vi "Expand Digital Pattern.vi"(5 "Zoom":refnum<vi>, 7 "Pattern Plot":refnum<vi>, 8 "error in (no error)":errorcluster, 9 "Select Patterns":i32[](array[numeric]), 10 "Rotations":u16, 11 "Patterns":T1[](array[typedef])) -> (0 "error out":errorcluster)   [LabVIEW 2017, in "Engine Simulation Toolkit System Explorer.lvlib"]
uses:
  Engine Simulation Toolkit System Explorer.lvlib
  Digital Pattern.ctl
  Digital Pattern Base.ctl
  Digital Pattern Remove Edge.ctl
  Digital Pattern Add Pulse.ctl
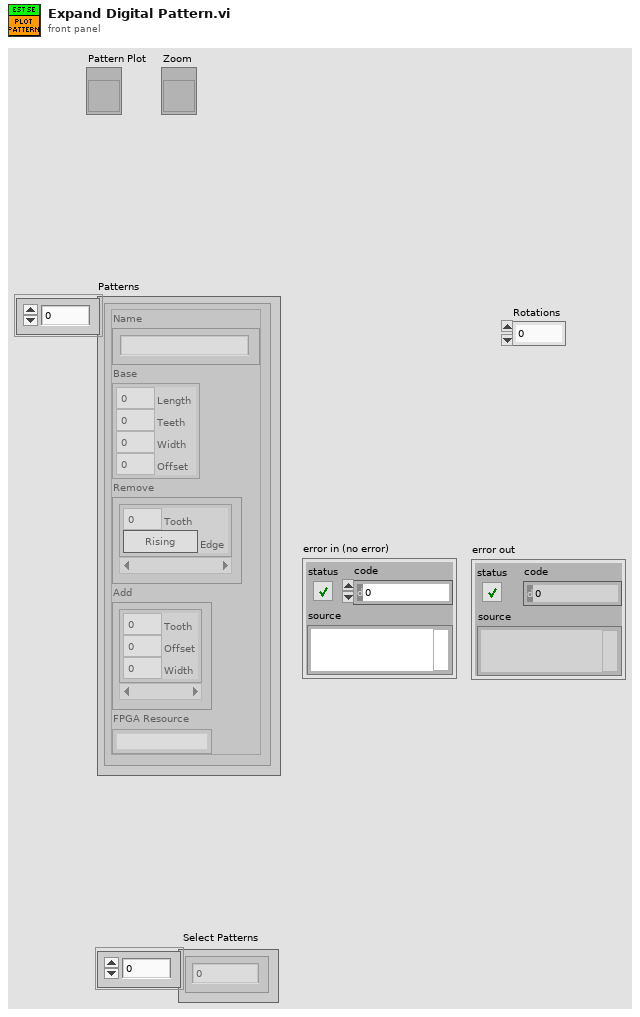
[diagram p1: front panel]
types:
  T1 = typedef "Engine Simulation Toolkit System Explorer.lvlib/Digital Pattern.ctl" = cluster{"Name":string, "Base":T2, "Remove":T3[], "Add":T4[], "FPGA Resource":string}
  T2 = typedef "Engine Simulation Toolkit System Explorer.lvlib/Digital Pattern Base.ctl" = cluster{"Length":dbl, "Teeth":u16, "Width":dbl, "Offset":dbl}
  T3 = typedef "Engine Simulation Toolkit System Explorer.lvlib/Digital Pattern Remove Edge.ctl" = cluster{"Tooth":u16, "Edge":bool}
  T4 = typedef "Engine Simulation Toolkit System Explorer.lvlib/Digital Pattern Add Pulse.ctl" = cluster{"Tooth":u16, "Offset":dbl, "Width":dbl}
  T5 = cluster{"Name":string, "Color":u32, "Style":u8, "Point Style":u8, "Name Visible":bool, "Allow Drag":bool, "Cursor Mode":u32, "Plot":i32, "Index":i32, "Position":cluster{"X":dbl, "Y":dbl}, "X Scale":u32, "Y Scale":u32, "Watch Plots":i32[], "Watch All Plots":bool, "Plot Area":i32, "Label Offset":cluster{"X":dbl, "Y":dbl}}
  T6 = cluster{"Name":string, "Color":u32, "Style":u8, "Point Style":u8, "Name Visible":bool, "Allow Drag":bool, "Cursor Mode":u32, "Plot":i32, "Index":i32, "Position":cluster{"X":dbl, "Y":dbl}, "X Scale":u32, "Y Scale":u32, "Watch Plots":i32[], "Watch All Plots":bool, "Plot Area":i32, "Label Offset":cluster{"X":dbl, "Y":dbl}}[]
  T7 = typedef "LVCursorListTypeDef.ctl" = cluster{"Name":string, "Color":u32, "Style":u8, "Point Style":u8, "Name Visible":bool, "Allow Drag":bool, "Cursor Mode":u32, "Plot":i32, "Index":i32, "Position":cluster{"X":dbl, "Y":dbl}, "X Scale":u32, "Y Scale":u32, "Watch Plots":i32[], "Watch All Plots":bool, "Plot Area":i32, "Label Offset":cluster{"X":dbl, "Y":dbl}}[]
  T8 = typedef "Engine Simulation Toolkit System Explorer.lvlib/Digital Pattern Expanded.ctl" = cluster{"X":dbl[], "Y":dbl[]}
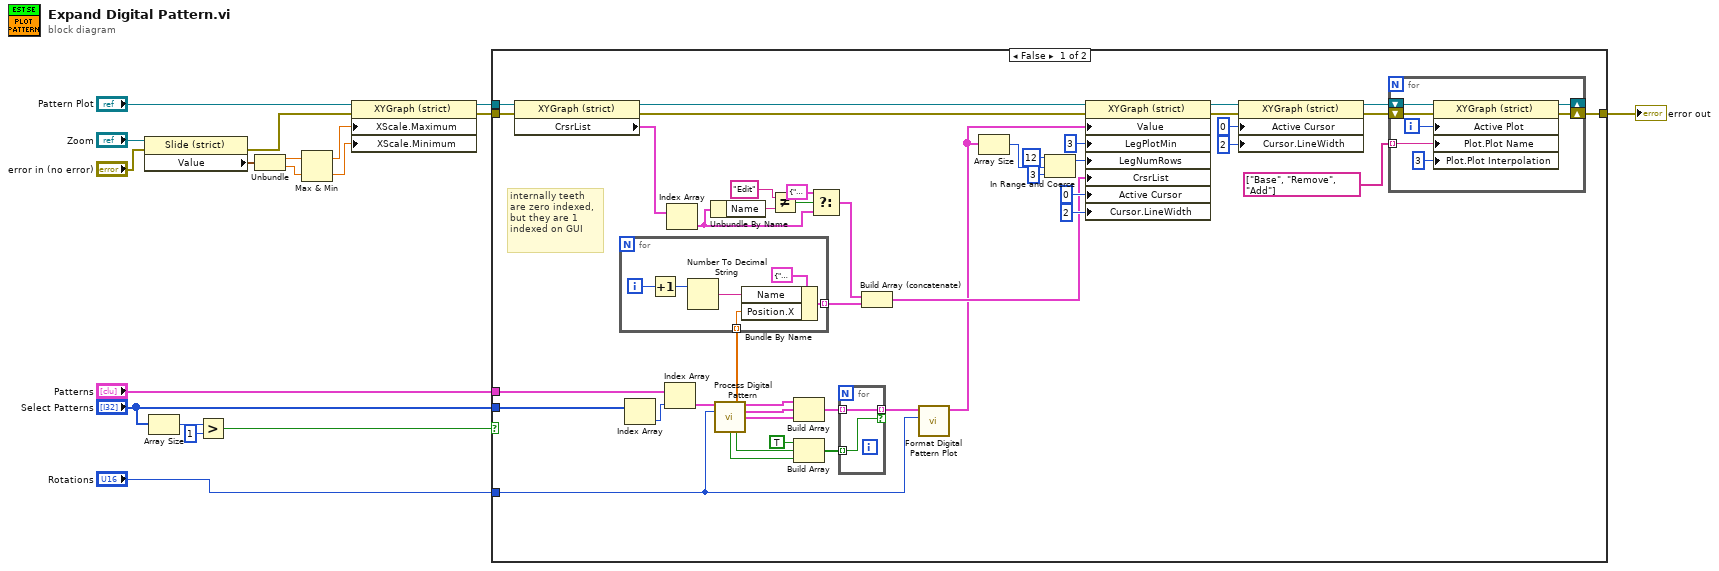
[diagram p0: block diagram]
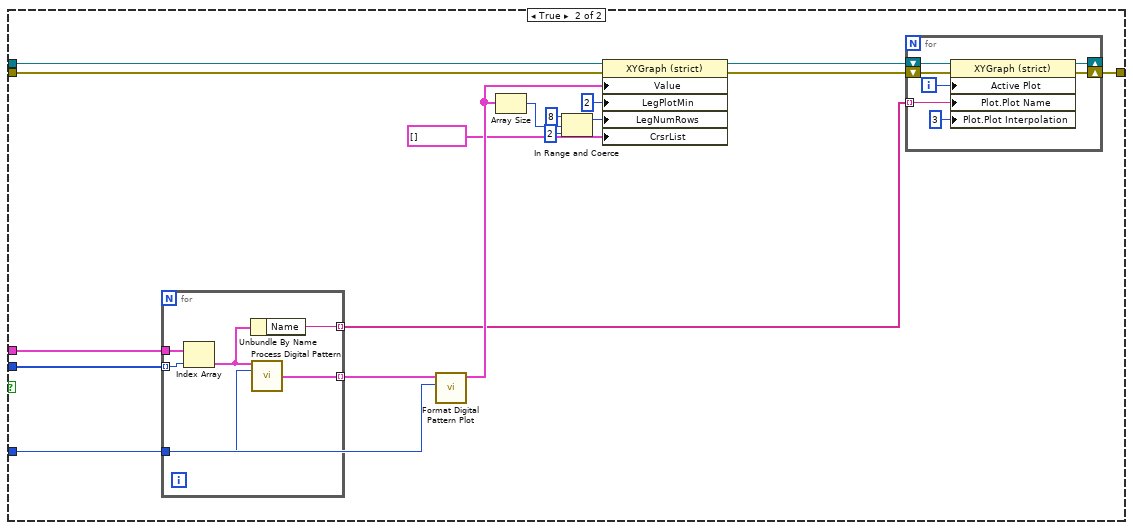
[diagram p2: hidden frame]
diagram:
  n1 = property class="Slide (strict)"(reference="Zoom", error in="error in (no error)") -> (error out=w3:errorcluster, "Value"=w16:cluster{dbl, dbl})  [unwired: 1 out]
  n2 = Array Size(array="Select Patterns") -> (size(s)=w11:i32)
  n3 = Greater?(x=w11, y=1) -> (0:w9:bool)
  n4 = Unbundle(w16) -> (w15:dbl, w12:dbl)
  n5 = Max & Min(x=w15, y=w12) -> (max(x,y)=w14:dbl, min(x,y)=w13:dbl)
  n6 = property class="XYGraph (strict)"(reference="Pattern Plot", error in=w3, "XScale.Maximum"=w14, "XScale.Minimum"=w13) -> (reference out=w6:refnum<vi>, error out=w2:errorcluster)
  n7 = case shown="False" w9 {
    tunnel: "Patterns" -> [w59 w86]
    tunnel: "Rotations" -> [w41 w88]
    tunnel: "Select Patterns" -> [w56 w85]
    tunnel: w6 -> [w47 w83]
    tunnel: w2 -> [w25 w81]
    tunnel: [w21 w79] -> w1
    frame False {
      # "internally teeth are zero indexed, but they are 1 indexed on GUI"
      n8 = property class="XYGraph (strict)"(reference=w47, error in=w25) -> (reference out=w46:refnum<vi>, error out=w24:errorcluster, "CrsrList"=w43:T7)
      n9 = Index Array(array=w56) -> (element=w57:i32)  [unwired: 1 in]
      n10 = Index Array(array=w59, index=w57) -> (element=w58:T1)
      n11 = Index Array(array=w43) -> (element=w27:T5)  [unwired: 1 in]
      n12 = Unbundle By Name(w27) -> ("Name"=w30:string)
      n13 = call "Process Digital Pattern.vi"("EPT Pattern"=w58, "Rotations"=w41) -> ("Base Teeth"=w26:dbl[], "Base"=w62:T8, 6:"Reduced"=w61:T8, 8:"Final"=w60:T8, 13:"Final"=w53:bool, 14:"Reduced"=w54:bool)  [unwired: 7 in, 1 out]
      n14 = for {
        tunnel: w26 -> [w74] mode=indexing
        tunnel: [w73] -> w50 mode=indexing
        i -> [w72]
        n15 = Increment(x=w72) -> (x+1=w70:i32)
        n16 = Number To Decimal String(number=w70) -> (decimal integer string=w75:string)  [unwired: 1 in]
        n17 = Bundle By Name(cluster=T5 {"Name"="", "Color"=0, "Style"=0, "Point Style"=0, "Name Visible"=TRUE, "Allow Drag"=FALSE, "Cursor Mode"=0, "Plot"=0, "Index"=0, "Position"={"X"=0.0, "Y"=0.0}, "X Scale"=0, "Y Scale"=0, "Watch Plots"=[], "Watch All Plots"=FALSE, "Plot Area"=0, "Label Offset"={"X"=0.0, "Y"=0.0}}, "Name"=w75, "Position.X"=w74) -> (w73:T5)
      }
      n18 = Not Equal?(x="Edit", y=w30) -> (x != y?=w28:bool)
      n19 = Build Array(w62, w61, w60) -> (w55:T8[])
      n20 = Build Array(TRUE ("element"), w54, w53) -> (w51:bool[])
      n21 = Select(t=T5 {"Name"="Edit", "Color"=0, "Style"=2, "Point Style"=13, "Name Visible"=TRUE, "Allow Drag"=TRUE, "Cursor Mode"=0, "Plot"=0, "Index"=26, "Position"={"X"=0.0, "Y"=1.0}, "X Scale"=0, "Y Scale"=0, "Watch Plots"=[], "Watch All Plots"=FALSE, "Plot Area"=0, "Label Offset"={"X"=0.0, "Y"=0.0}} ("element"), s=w28, f=w27) -> (s? t:f=w48:T5)
      n22 = for {
        tunnel: w55 -> [w77] mode=indexing
        tunnel: [w77] -> w40 mode=indexing if=w76
        tunnel: w51 -> [w76] mode=indexing
      }
      n23 = Build Array (concatenate)(w48, w50) -> (w42:T6)
      n24 = call "Format Digital Pattern Plot.vi"("Rotations"=w41, "Patterns"=w40) -> ("Patterns"=w35:T8[])  [unwired: 9 in]
      n25 = Array Size(array=w35) -> (size(s)=w36:i32)
      n26 = In Range and Coerce(upper limit=12, x=w36, lower limit=3) -> (coerced(x)=w37:i32)  [unwired: 1 out]
      n27 = property class="XYGraph (strict)"(reference=w46, error in=w24, "Value"=w35, "LegPlotMin"=u32 3 ("Legend:Plot Minimum"), "LegNumRows"=w37, "CrsrList"=w42, "Active Cursor"=u32 0, "Cursor.LineWidth"=u8 2 ("Cursor.Line Width")) -> (reference out=w34:refnum<vi>, error out=w23:errorcluster)
      n28 = property class="XYGraph (strict)"(reference=w34, error in=w23, "Active Cursor"=u32 0, "Cursor.LineWidth"=u8 2 ("Cursor.Line Width")) -> (reference out=w33:refnum<vi>, error out=w22:errorcluster)
      n29 = for {
        shift-right: [w68] -> _
        shift-left: w33 -> [w69]
        tunnel: string[] ["Base", "Remove", "Add"] -> [w66] mode=indexing
        shift-right: [w63] -> w21
        shift-left: w22 -> [w64]
        i -> [w67]
        n30 = property class="XYGraph (strict)"(reference=w69, error in=w64, "Active Plot"=w67, "Plot.Plot Name"=w66, "Plot.Plot Interpolation"=u8 3) -> (reference out=w68:refnum<vi>, error out=w63:errorcluster)
      }
    }
    frame True {
      n31 = for {
        tunnel: [w95] -> w89 mode=indexing
        tunnel: w86 -> [w100]
        tunnel: w85 -> [w99] mode=indexing
        tunnel: w88 -> [w98]
        tunnel: [w96] -> w87 mode=indexing
        n32 = Index Array(array=w100, index=w99) -> (element=w97:T1)
        n33 = Unbundle By Name(w97) -> ("Name"=w96:string)
        n34 = call "Process Digital Pattern.vi"("EPT Pattern"=w97, "Rotations"=w98) -> ("Final"=w95:T8)  [unwired: 7 in, 6 out]
      }
      n35 = call "Format Digital Pattern Plot.vi"("Rotations"=w88, "Patterns"=w89) -> ("Patterns"=w90:T8[])  [unwired: 9 in]
      n36 = Array Size(array=w90) -> (size(s)=w91:i32)
      n37 = In Range and Coerce(upper limit=8, x=w91, lower limit=2) -> (coerced(x)=w92:i32)  [unwired: 1 out]
      n38 = property class="XYGraph (strict)"(reference=w83, error in=w81, "Value"=w90, "LegPlotMin"=u32 2 ("Legend:Plot Minimum"), "LegNumRows"=w92, "CrsrList"=T6 [] ("Cursor List")) -> (reference out=w82:refnum<vi>, error out=w80:errorcluster)
      n39 = for {
        shift-right: [w106] -> _
        shift-left: w82 -> [w107]
        tunnel: w87 -> [w104] mode=indexing
        shift-right: [w101] -> w79
        shift-left: w80 -> [w102]
        i -> [w105]
        n40 = property class="XYGraph (strict)"(reference=w107, error in=w102, "Active Plot"=w105, "Plot.Plot Name"=w104, "Plot.Plot Interpolation"=u8 3) -> (reference out=w106:refnum<vi>, error out=w101:errorcluster)
      }
    }
  }
  "error out" <- w1
